vi "Output_waveform_and_triggers.vi"() -> ()   [LabVIEW 2019]
uses:
  Create_waveform/build_waveform.lvclass
  Combine_pulses/Combine_pulses.lvclass
  Write_to_file/Write_to_file.lvclass
  Plot_waveform/Plot_waveform.lvclass
panel:
  in  "Create Trigger?":bool
  in  "Pretrigger (points)":dbl
  out "Padded waveform":waveform(dbl)[](graph)
  out "Waveform":waveform(dbl)(graph)
  in  "start path":path=path "C:/GitHub/PulseEcho/PulsedFieldEcho"
  in  "Repetition frequency":dbl=20000.0
  in  "Pulse Duraction":dbl=0.01
  in  "standard deviation":dbl=0.1
  in  "NWaves":i32=10
  in  "Frequency":dbl=220000000.0
  in  "clock rate":dbl=1200000000.0
  # "Pulse Parameters"
  # "Select Path"
  # "Waveform Parameters"
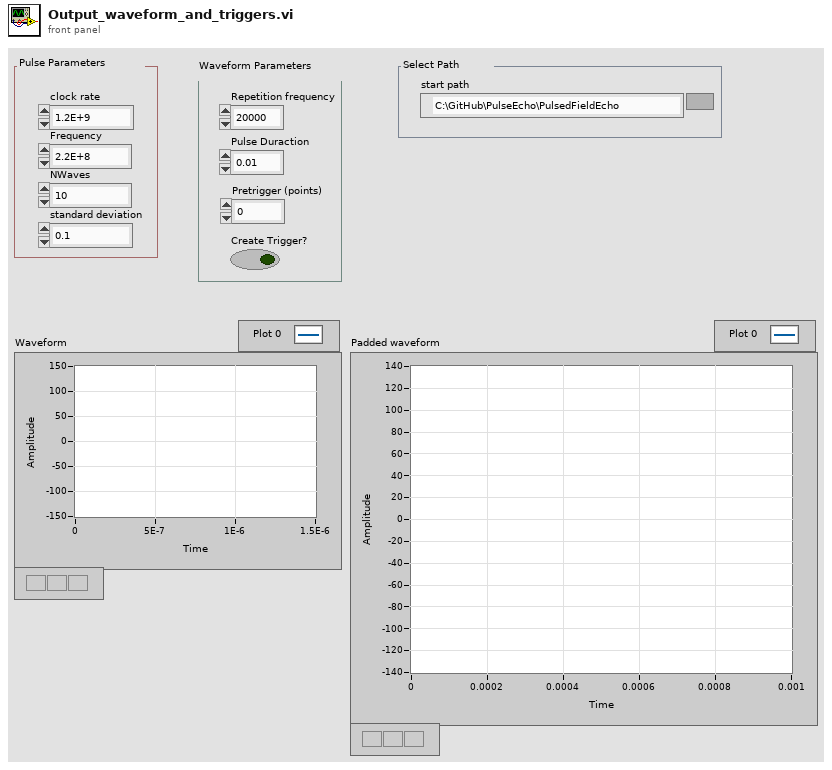
[diagram p1: front panel]
types:
  T1 = enum16{"open", "replace", "create", "open or create", "replace or create", "replace or create with confirmation"}
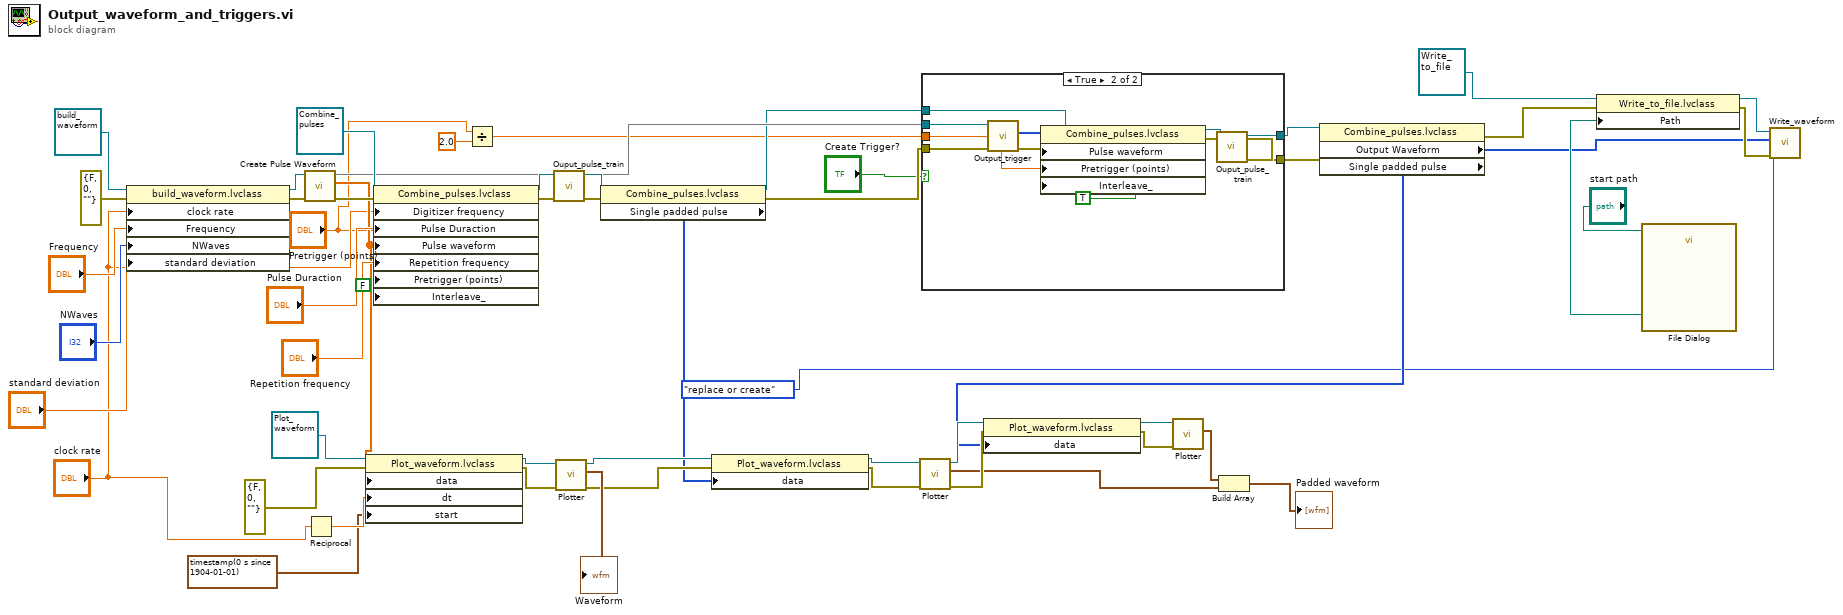
[diagram p0: block diagram]
diagram:
  n1 = property class="build_waveform.lvclass"(reference=refnum<class "build_waveform.lvclass"> refnum ("build_waveform.lvclass"), error in=errorcluster {"status"=FALSE, "code"=0, "source"=""} ("error in (no error)"), "clock rate"="clock rate", "Frequency"="Frequency", "NWaves"="NWaves", "standard deviation"="standard deviation") -> (reference out=w50:refnum<class "build_waveform.lvclass">, error out=w49:errorcluster)
  n2 = call "Create Pulse Waveform.vi"("error in (no error)"=w49, "Waveform parameters"=w50) -> ("error out"=w47:errorcluster, "Signal"=w36:dbl[], 3:w23)  [unwired: 6 in, 1 out]
  n3 = Reciprocal(x="clock rate") -> (1/x=w37:dbl)
  n4 = property class="Plot_waveform.lvclass"(reference=refnum<class "Plot_waveform.lvclass"> refnum ("Plot_waveform.lvclass"), error in=errorcluster {"status"=FALSE, "code"=0, "source"=""} ("error in (no error)"), "data"=w36, "dt"=w37, "start"=timestamp(0 s since 1904-01-01)) -> (reference out=w34:refnum<class "Plot_waveform.lvclass">, error out=w33:errorcluster)
  n5 = property class="Combine_pulses.lvclass"(reference=refnum<class "Combine_pulses.lvclass"> refnum ("Combine_pulses.lvclass"), error in=w47, "Digitizer frequency"="clock rate", "Pulse Duraction"="Pulse Duraction", "Pulse waveform"=w36, "Repetition frequency"="Repetition frequency", "Pretrigger (points)"="Pretrigger (points)", "Interleave_"=FALSE) -> (reference out=w26:refnum<class "Combine_pulses.lvclass">, error out=w44:errorcluster)
  n6 = Divide(x="Pretrigger (points)", y=2.0) -> (x/y=w21:dbl)
  n7 = call-dynamic "Ouput_pulse_train.vi"("error in (no error)"=w44, "Combine_pulses in"=w26) -> ("error out"=w42:errorcluster, "Combine_pulses out"=w43:refnum<class "Combine_pulses.lvclass">)  [unwired: 8 in]
  n8 = call-dynamic "Plotter.vi"("error in (no error)"=w33, "Plot_waveform in"=w34) -> ("error out"=w30:errorcluster, "output waveform"=→"Waveform":waveform(dbl), "Plot_waveform out"=w31:refnum<class "Plot_waveform.lvclass">)  [unwired: 7 in]
  n9 = property class="Combine_pulses.lvclass"(reference=w43, error in=w42) -> (reference out=w22:refnum<class "Combine_pulses.lvclass">, error out=w7:errorcluster, "Single padded pulse"=w29:i8[])
  n10 = property class="Plot_waveform.lvclass"(reference=w31, error in=w30, "data"=w29) -> (reference out=w28:refnum<class "Plot_waveform.lvclass">, error out=w27:errorcluster)
  n11 = call-dynamic "Plotter.vi"("error in (no error)"=w27, "Plot_waveform in"=w28) -> ("error out"=w17:errorcluster, "output waveform"=w12:waveform(dbl), "Plot_waveform out"=w18:refnum<class "Plot_waveform.lvclass">)  [unwired: 7 in]
  n12 = case shown="True" "Create Trigger?" {
    tunnel: w23 -> [_ w68]
    tunnel: w22 -> [w57 w67]
    tunnel: w21 -> [_ w65]
    tunnel: [w57 w61] -> w20
    tunnel: [w56 w60] -> w19
    tunnel: w7 -> [w56 w58]
    frame False {
    }
    frame True {
      n13 = call-dynamic "Output_trigger.vi"("error in (no error)"=w58, "build_waveform in"=w68) -> ("error out"=w66:errorcluster, "Array"=w64:i8[])  [unwired: 7 in, 1 out]
      n14 = property class="Combine_pulses.lvclass"(reference=w67, error in=w66, "Pulse waveform"=w64, "Pretrigger (points)"=w65, "Interleave_"=TRUE) -> (reference out=w63:refnum<class "Combine_pulses.lvclass">, error out=w62:errorcluster)
      n15 = call-dynamic "Ouput_pulse_train.vi"("error in (no error)"=w62, "Combine_pulses in"=w63) -> ("error out"=w60:errorcluster, "Combine_pulses out"=w61:refnum<class "Combine_pulses.lvclass">)  [unwired: 8 in]
    }
  }
  n16 = property class="Combine_pulses.lvclass"(reference=w20, error in=w19) -> (error out=w6:errorcluster, "Output Waveform"=w2:i8[], "Single padded pulse"=w16:i8[])  [unwired: 1 out]
  n17 = property class="Plot_waveform.lvclass"(reference=w18, error in=w17, "data"=w16) -> (reference out=w15:refnum<class "Plot_waveform.lvclass">, error out=w14:errorcluster)
  n18 = call-dynamic "Plotter.vi"("error in (no error)"=w14, "Plot_waveform in"=w15) -> ("output waveform"=w13:waveform(dbl))  [unwired: 7 in, 2 out]
  n19 = Build Array(w13, w12) -> (→"Padded waveform":waveform(dbl)[])
  n20 = call "File Dialog"("start path"="start path") -> ("selected path"=w41:path)  [unwired: 11 in, 3 out]
  n21 = property class="Write_to_file.lvclass"(reference=refnum<class "Write_to_file.lvclass"> refnum ("Write_to_file.lvclass"), error in=w6, "Path"=w41) -> (reference out=w3:refnum<class "Write_to_file.lvclass">, error out=w5:errorcluster)
  n22 = call-dynamic "Write_waveform.vi"("error in (no error)"=w5, "operation (0:open)"=T1."replace or create", "Signal"=w2, "Write_to_file in"=w3) -> ()  [unwired: 6 in, 2 out]
